vi "S2DS_Export data (SubVI).vi"(8 "error in (no error)":errorcluster, 10 "Data in":dbl[](array[numeric]), 11 "connection id":refnum<k13>) -> (0 "error out":errorcluster, 3 "connection out":refnum<k13>)   [LabVIEW 2025]
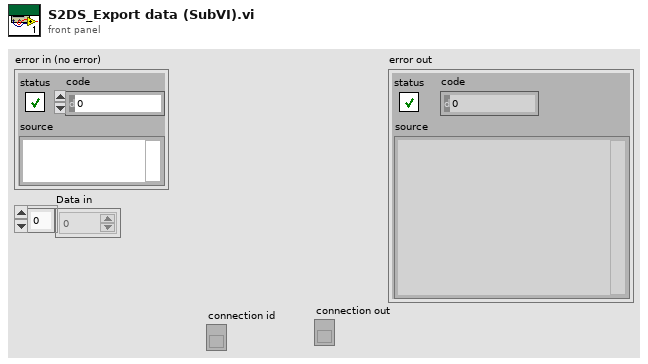
[diagram p1: front panel]
types:
  T1 = enum16{"Read", "Write", "ReadWrite", "BufferedRead", "BufferedReadWrite"}
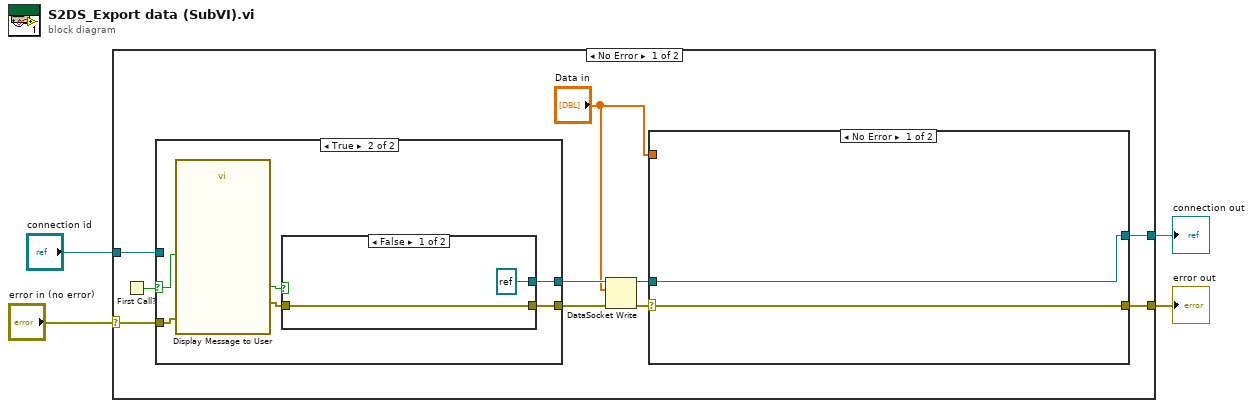
[diagram p0: block diagram]
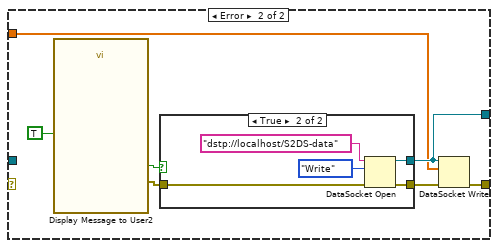
[diagram p2: hidden frame]
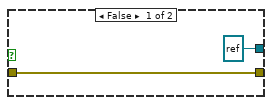
[diagram p3: hidden frame]
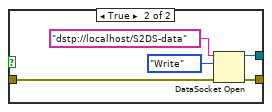
[diagram p5: hidden frame]
diagram:
  n1 = case shown="No Error" "error in (no error)" {
    selector: "error in (no error)" -> [w5 w47]
    tunnel: "connection id" -> [w12 w46]
    tunnel: [w8 w47] -> w3
    tunnel: [w6 w46] -> w2
    frame No Error {
      n2 = First Call?() -> (First Call?: T/F=w11:bool)
      n3 = case shown="True" w11 {
        selector: w11 -> [_ w38]
        tunnel: [w32 w35] -> w14
        tunnel: [w31 w34] -> w13
        tunnel: w12 -> [w32 _]
        tunnel: w5 -> [w31 w33]
        frame False {
        }
        frame True {
          n4 = call "Display Message to User"("error in (no error)"=w33, "Enable"=w38) -> ("error out"=w36:errorcluster, "OK"=w37:bool)  [unwired: 8 in]
          n5 = case shown="False" w37 {
            tunnel: w36 -> [w39 w43]
            tunnel: [refnum<k13> refnum ("connection id") w42] -> w35
            tunnel: [w39 w41] -> w34
            frame False {
            }
            frame True {
              n6 = DataSocket Open(8:w43, 10:T1."Write" ("mode"), 11:"dstp://localhost/S2DS-data" ("Write Location")) -> (0:w41:errorcluster, 3:w42:refnum<k13>)  [unwired: 1 in]
            }
          }
        }
      }
      n7 = DataSocket Write(8:w13, 10:"Data in", 11:w14) -> (0:w10:errorcluster, 3:w7:refnum<k13>)  [unwired: 1 in, 1 out]
      n8 = case shown="No Error" w10 {
        selector: w10 -> [w16 _]
        tunnel: [w15 w20] -> w6
        tunnel: "Data in" -> [_ w18]
        tunnel: [w16 w17] -> w8
        tunnel: w7 -> [w15 _]
        frame No Error {
        }
        frame Error {
          n9 = call "Display Message to User2"("Enable"=TRUE) -> ("error out"=w22:errorcluster, "OK"=w23:bool)  [unwired: 9 in]
          n10 = case shown="True" w23 {
            tunnel: w22 -> [w24 w28]
            tunnel: [refnum<k13> refnum ("connection id") w27] -> w20
            tunnel: [w24 w26] -> w19
            frame False {
            }
            frame True {
              n11 = DataSocket Open(8:w28, 10:T1."Write" ("mode"), 11:"dstp://localhost/S2DS-data" ("Write Location")) -> (0:w26:errorcluster, 3:w27:refnum<k13>)  [unwired: 1 in]
            }
          }
          n12 = DataSocket Write(8:w19, 10:w18, 11:w20) -> (0:w17:errorcluster)  [unwired: 1 in, 2 out]
        }
      }
    }
    frame Error {
    }
  }
  "error out" <- w3
  "connection out" <- w2
